vi "2100_Hybrid_ODFT_Meas.vi"(0 "Semiconductor Module Context":T5, 1 "USID":T4 max=15, 2 "Script Name":string="IVIOKGD", 3 "Publishable IDs":string[](array[string])=["LowPower", "Active"], 5 "All_Scripts":string[][](array[string]), 7 "SMU_Pins":string[](array[string])=["VSU"], 9 "HSDIO_Pins":string[](array[string])=["CLK", "SDA"], 11 "Error In":errorcluster, 12 "Master_Register_Data_Array_In":T2 {"Address" format="%.0x"}, 13 "PI_1_Meas":dbl format="%#_6p") -> (15 "Error Out":errorcluster)   [LabVIEW 2013]
uses:
  Controls/USID.ctl
  <vilib>/NI_TestStand_SemiconductorModule/NI_TestStand_Semiconductor_Module.lvlibp/PinMap/General/SemiconductorModuleContext.ctl
  Controls/Master_Reg_Data_Array.ctl
  Controls/Reg_Address_Data.ctl
  <vilib>/NI_TestStand_SemiconductorModule/NI_TestStand_Semiconductor_Module.lvlibp/PinMap/DC Power/PinsToNIDCPowerSessions.vi
  <vilib>/NI_TestStand_SemiconductorModule/NI_TestStand_Semiconductor_Module.lvlibp/PinMap/Deprecated/PublishDataDoubleMultiplePinsMultipleInstruments.vi
  <vilib>/NI_TestStand_SemiconductorModule/NI_TestStand_Semiconductor_Module.lvlibp/PinMap/Deprecated/PublishDataDoubleMultiplePinsSingleInstrument.vi
  <vilib>/NI_TestStand_SemiconductorModule/NI_TestStand_Semiconductor_Module.lvlibp
panel:
  out "iPI_Calc":dbl[](array[numeric])
  in  "Tab Control":T1(tab)
  out "current measurements":dbl[][](array[numeric])
  out "Delta_iHV_Measurements":dbl[][](array[numeric])
  out "Master_Register_Data_Array_Out":T2 {"Address" format="%.0x"}
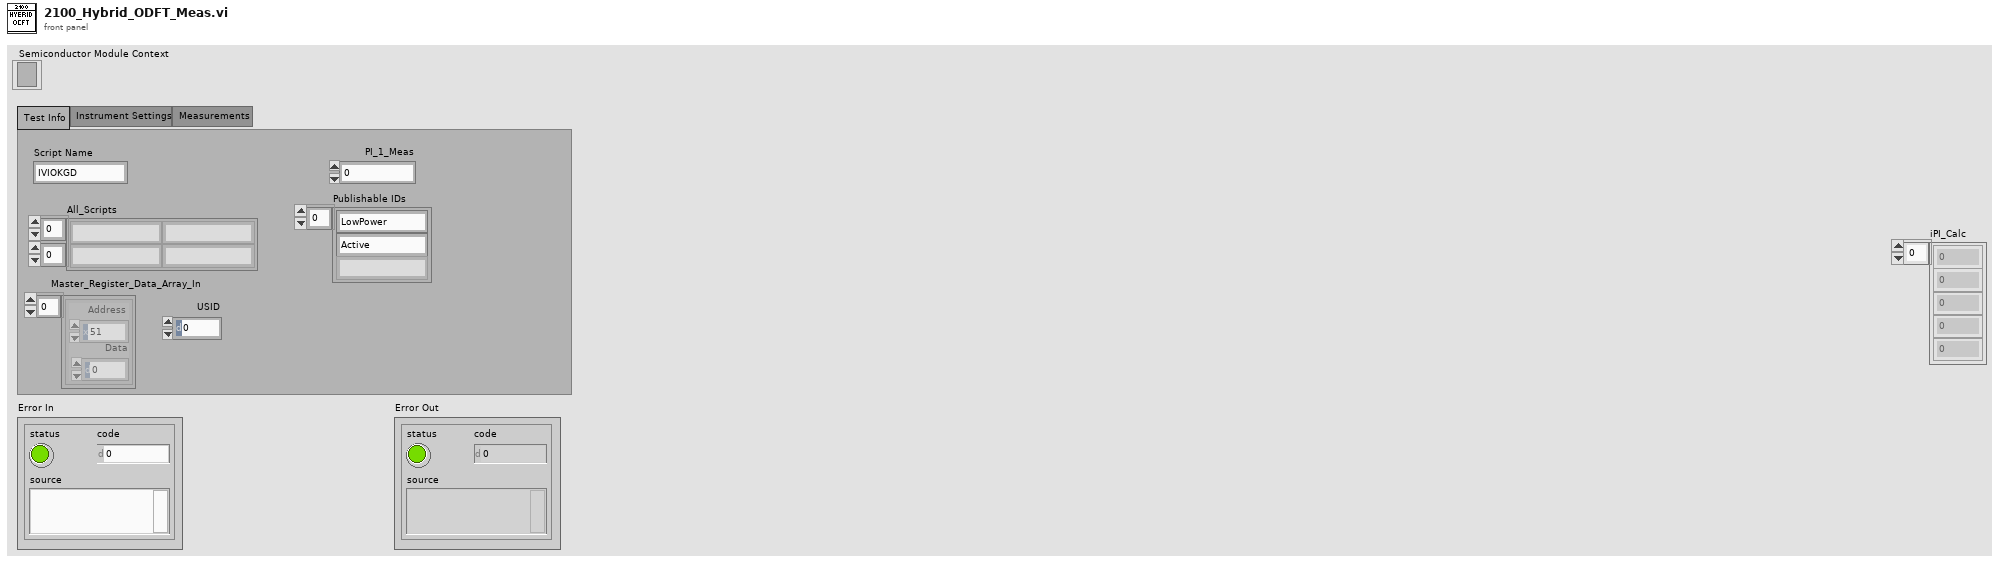
[diagram p1: front panel]
types:
  T1 = enum32{"Test Info", "Instrument Settings", "Measurements"}
  T2 = typedef "Master_Reg_Data_Array.ctl" = T3[]
  T3 = typedef "Reg_Address_Data.ctl" = cluster{"Address":u8, "Data":u8}
  T4 = typedef "USID.ctl" = u8
  T5 = typedef "NI_TestStand_Semiconductor_Module.lvlibp/SemiconductorModuleContext.ctl" = refnum<k7>
  T6 = typedef "Script Functions_Array.ctl" = enum16{"Reg_Write", "Bit_Write", "Delay", "Read"}[]
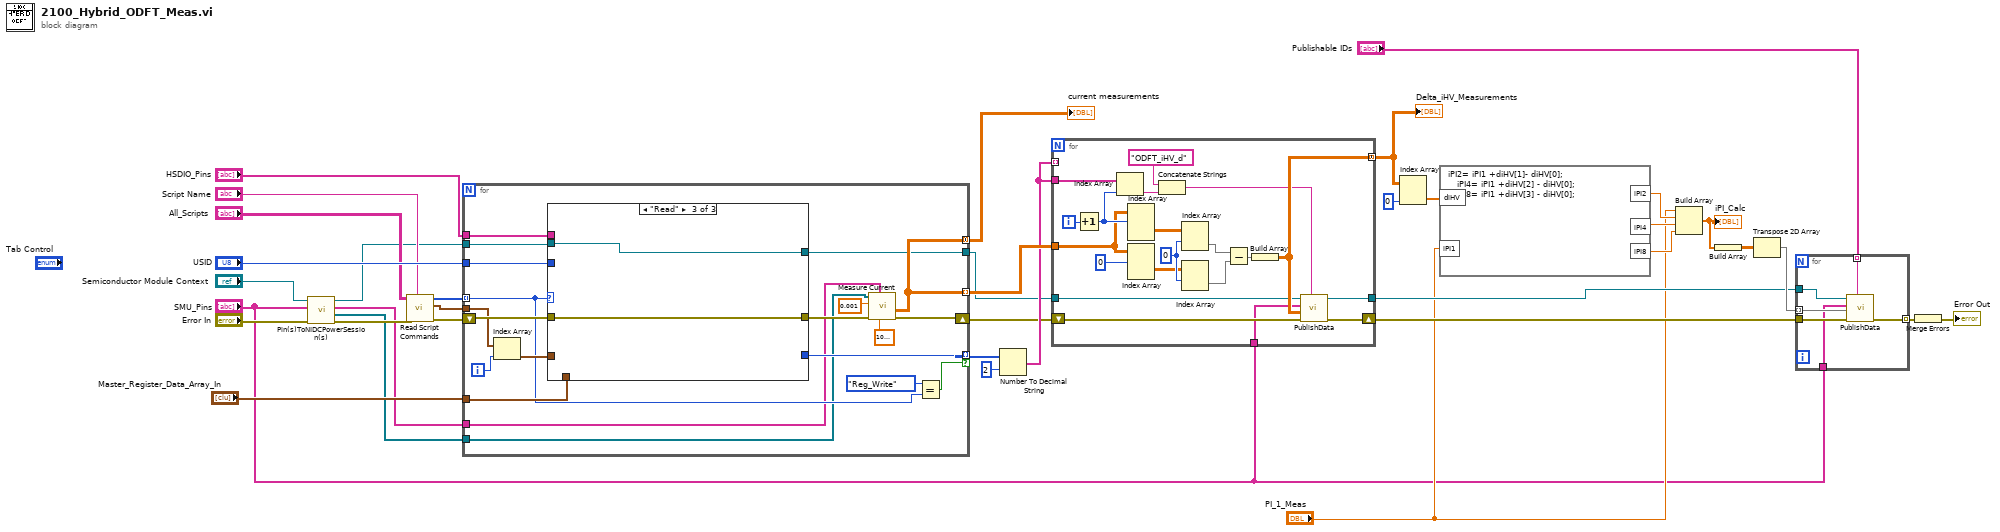
[diagram p0: block diagram]
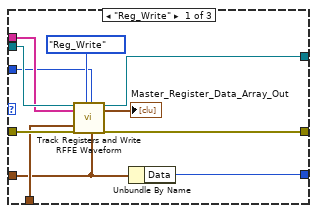
[diagram p2: hidden frame]
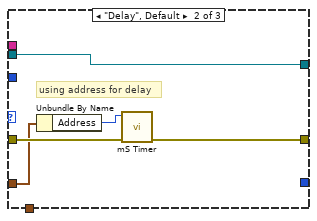
[diagram p3: hidden frame]
diagram:
  n1 = call-poly <vilib>:"Pin(s)ToNIDCPowerSession(s).vi"("error in (no error)"="Error In", "Pins"="SMU_Pins", "Semiconductor Module Context"="Semiconductor Module Context") -> ("error out"=w9:errorcluster, "Instrument Sessions"=w8:refnum<k15>[], "Channel Lists"=w7:string[], "Semiconductor Module Context Out"=w10:T5)  [unwired: 4 in, 1 out]
  n2 = call "Read Script Commands.vi"("Test Name"="Script Name", "Error In"=w9, "All_Scripts"="All_Scripts") -> ("Error Out"=w32:errorcluster, "Script_Data"=w33:T3[], "Script_Functions"=w34:T6)  [unwired: 6 in]
  n3 = for {
    tunnel: "USID" -> [w56]
    tunnel: w34 -> [w42] mode=indexing
    tunnel: w33 -> [w53]
    tunnel: w10 -> [w55]
    tunnel: "HSDIO_Pins" -> [w54]
    shift-right: [w46] -> w24
    shift-left: w32 -> [w57]
    tunnel: "Master_Register_Data_Array_In" -> [w50]
    tunnel: [w45] -> w29 mode=indexing
    tunnel: [w45] -> w26 mode=concatenating
    tunnel: [w44] -> w28 mode=indexing if=w41
    tunnel: w8 -> [w40]
    tunnel: w7 -> [w39]
    tunnel: [w38] -> w6
    i -> [w51]
    n4 = Index Array(array=w53, index=w51) -> (element=w52:T3)
    n5 = case shown="\"Read\"" w42 {
      tunnel: w52 -> [w59 w72 _]
      tunnel: w57 -> [w68 w73 w75]
      tunnel: w56 -> [w60 _ _]
      tunnel: w55 -> [w66 w69 w74]
      tunnel: w54 -> [w64 _ _]
      tunnel: [w67 w70 w75] -> w47
      tunnel: [w65 w69 w74] -> w38
      tunnel: w50 -> [w62 _ _]
      tunnel: [w58 _ _] -> w44
      frame "Reg_Write" {
        n6 = call "Track Registers and Write RFFE Waveform.vi"("Semiconductor Module Context"=w66, "Pins"=w64, "Master_Register_Data_Array_In"=w62, "Error In"=w68, "Script_Functions"=enum16{"Reg_Write", "Bit_Write"}."Reg_Write", "USID"=w60, "Reg_Address_Data"=w59) -> ("Semiconductor Module Context Out"=w65:T5, "Master_Register_Data_Array_Out"=→"Master_Register_Data_Array_Out":T2, "Error Out"=w67:errorcluster)  [unwired: 10 in]
        n7 = Unbundle By Name(w59) -> ("Data"=w58:u8)
      }
      frame "Delay", Default {
        # "using address for delay"
        n8 = Unbundle By Name(w72) -> ("Address"=w71:u8)
        n9 = call "mS Timer.vi"("Error In"=w73, "Delay(S)"=w71) -> ("Error Out"=w70:errorcluster)  [unwired: 9 in]
      }
      frame "Read" {
      }
    }
    n10 = call "Measure Current.vi"("Result Multiplier"=1000000.0, "Channel Lists"=w39, "error in (no error)"=w47, "Delay Time (s)"=0.001 ("Result Multiplier"), "DCPower Sessions In"=w40) -> ("error out"=w46:errorcluster, "current measurements"=w45:dbl[][])  [unwired: 4 in, 1 out]
    n11 = Equal?(x=enum16{"Reg_Write", "Bit_Write"}."Reg_Write" ("Script_Functions"), y=w42) -> (x = y?=w41:bool)
  }
  "current measurements" <- w26
  n12 = Number To Decimal String(number=w28, width (-)=i16 2) -> (decimal integer string=w25:string[])
  n13 = for {
    shift-right: [w84] -> w5
    shift-left: w24 -> [w83]
    tunnel: w29 -> [w90]
    tunnel: [w82] -> w16 mode=concatenating
    tunnel: w25 -> [w80]
    tunnel: w25 -> [_] mode=indexing
    tunnel: w6 -> [w78]
    tunnel: "SMU_Pins" -> [w77]
    tunnel: [w76] -> w3
    i -> [w94]
    w91 = 0 ("index (page)")
    n14 = Increment(x=w94) -> (x+1=w92:i32)
    n15 = Index Array(array=w80, index=w92) -> (element=w79:string)
    n16 = Index Array(array=w90, index (dim 0)=w92) -> (element=w89:dbl[][])  [unwired: 2 in]
    n17 = Index Array(array=w90, index (dim 0)=0 ("index (page)")) -> (element=w88:dbl[][])  [unwired: 2 in]
    n18 = Concatenate Strings("ODFT_iHV_d", w79) -> (w81:string)
    n19 = Index Array(array=w89, index (row)=w91) -> (element=w86:dbl[])  [unwired: 1 in]
    n20 = Index Array(array=w88, index (row)=w91) -> (element=w87:dbl[])  [unwired: 1 in]
    n21 = Subtract(x=w86, y=w87) -> (x-y=w85:dbl[])
    n22 = Build Array(w85) -> (w82:dbl[][])
    n23 = call-poly <vilib>:"PublishData.vi"("Measurement Id"=w81, "error in (no error)"=w83, "Data In"=w82, "Pins"=w77, "Semiconductor Module Context"=w78) -> ("error out"=w84:errorcluster, "Semiconductor Module Context Out"=w76:T5)  [unwired: 5 in]
  }
  "Delta_iHV_Measurements" <- w16
  n24 = Index Array(array=w16, index (col)=0 ("disabled index (col)")) -> (element=w22:dbl[])  [unwired: 1 in]
  n25 = formula code="iPI2= iPI1 +diHV[1]- diHV[0];\n   iPI4= iPI1 +diHV[2] - diHV[0];\n   iPI8= iPI1 +diHV[3] - diHV[0];"("diHV"=w22, "iPI1"="PI_1_Meas") -> ("iPI2"=w19:dbl, "iPI4"=w18:dbl, "iPI8"=w17:dbl)
  n26 = Build Array("PI_1_Meas", w19, w18, w17) -> (w21:dbl[])
  "iPI_Calc" <- w21
  n27 = Build Array(w21) -> (w20:dbl[][])
  n28 = Transpose 2D Array(2D array=w20) -> (transposed array=w14:dbl[][])
  n29 = for {
    tunnel: [w101] -> w15 mode=indexing
    tunnel: w14 -> [w100] mode=indexing
    tunnel: "Publishable IDs" -> [w99] mode=indexing
    tunnel: w5 -> [w98]
    tunnel: w3 -> [w97]
    tunnel: "SMU_Pins" -> [w96]
    n30 = call-poly <vilib>:"PublishData.vi"("Measurement Id"=w99, "error in (no error)"=w98, "Data In"=w100, "Pins"=w96, "Semiconductor Module Context"=w97) -> ("error out"=w101:errorcluster)  [unwired: 5 in, 1 out]
  }
  n31 = Merge Errors(w15) -> (→"Error Out":errorcluster)
